vi "obtenerPruebas.vi"(8 "error in (no error)":errorcluster, 11 "Equipo in":refnum<class "Fabrica de Equipos.lvclass">) -> (0 "error out":errorcluster, 2 "Equipo.lvclass":refnum<class "Equipo.lvclass">, 3 "Equipo out":refnum<class "Fabrica de Equipos.lvclass">)   [LabVIEW 2019, in "Fabrica de Equipos.lvclass"]
uses:
  Fabrica de Equipos.lvclass
  Equipo/Equipo.lvclass
  Fabrica de Equipos.lvclass/Fabrica de Equipos.ctl
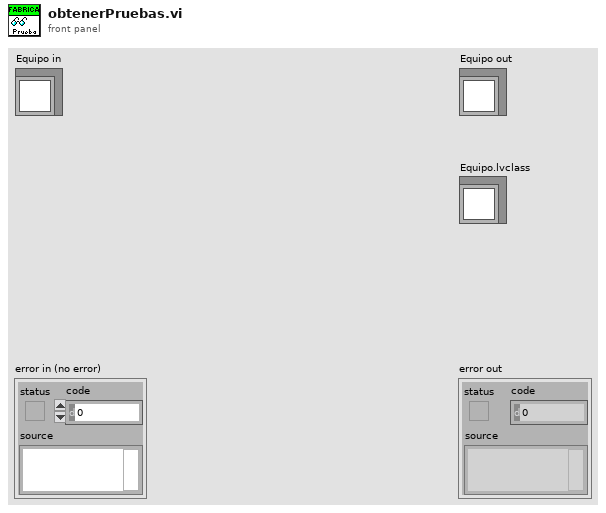
[diagram p1: front panel]
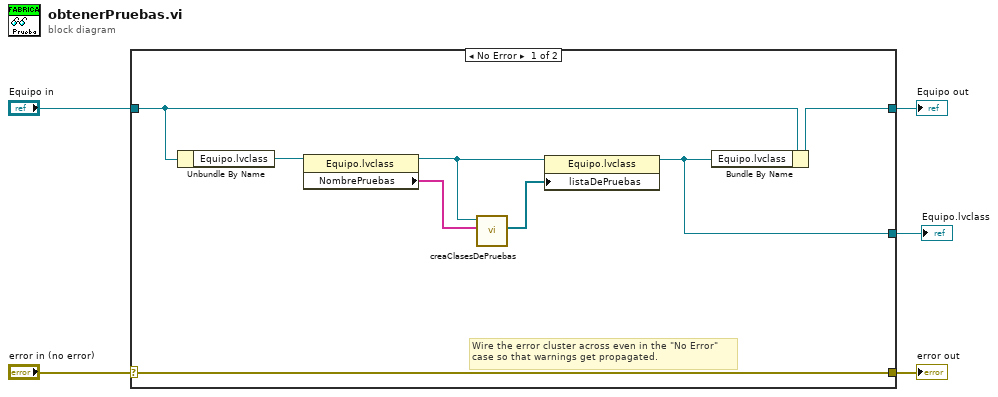
[diagram p0: block diagram]
diagram:
  n1 = case shown="No Error" "error in (no error)" {
    selector: "error in (no error)" -> [w13 w15]
    tunnel: [w13 w15] -> w4
    tunnel: [w11 w14] -> w3
    tunnel: "Equipo in" -> [w12 w14]
    tunnel: [w10 _] -> w2
    frame No Error {
      # "Wire the error cluster across even in the \"No Error\"\ncase so that warnings get propagated."
      n2 = Unbundle By Name(w12) -> ("Equipo.lvclass"=w8:refnum<class "Equipo.lvclass">)
      n3 = property class="Equipo.lvclass"(reference=w8) -> (reference out=w7:refnum<class "Equipo.lvclass">, "NombrePruebas"=w6:string[])  [unwired: 1 in, 1 out]
      n4 = call-dynamic "creaClasesDePruebas.vi"("NombrePruebas"=w6, "Equipo in"=w7) -> ("listaDePruebas"=w9:refnum<class "Prueba.lvclass">[])  [unwired: 7 in, 2 out]
      n5 = property class="Equipo.lvclass"(reference=w7, "listaDePruebas"=w9) -> (reference out=w10:refnum<class "Equipo.lvclass">)  [unwired: 1 in, 1 out]
      n6 = Bundle By Name(cluster=w12, "Equipo.lvclass"=w10) -> (w11:refnum<class "Fabrica de Equipos.lvclass">)
    }
    frame Error {
    }
  }
  "error out" <- w4
  "Equipo out" <- w3
  "Equipo.lvclass" <- w2
